vi "validate.vi"(8 "error in":errorcluster, 11 "Digitizer configuration":refnum<class "Digitizer configuration.lvclass">) -> (0 "error out":errorcluster, 3 "Digitizer configuration out":refnum<class "Digitizer configuration.lvclass">)   [LabVIEW 2025, in "Digitizer.lvlib" / "Digitizer configuration.lvclass"]
doc: "Provides an interface for performing validation on a given configuration. Any children should define the behavior of this function to ensure that the configuration in memory can be used by the runtime class.Copyright 2017 National Instruments Corporation\n\nLicensed under the Apache License, Version 2.0 (the \"License\"); you may not use this file except in compliance with the License. You may obtain a copy of the License at http://www.apache.org/licenses/LICENSE-2.0\nUnless required by applicable law or agreed to in writing, software distributed under the License is distributed on an \"AS IS\" BASIS, WITHOUT WARRANTIES OR CONDITIONS OF ANY KIND, either express or implied. See the License for the specific language governing permissions and limitations under the License."
uses:
  Digitizer configuration.lvclass
  Users/Public/Documents/Sandia National Labs/TSS Plugin/Abstract Engine.lvlibp/Plugin/Abstract/Instrument configuration/Read Instrument Setting.vi
  Digitizer configuration.lvclass/Digitizer configuration.ctl
  Users/Public/Documents/Sandia National Labs/TSS Plugin/CEF.lvlibp
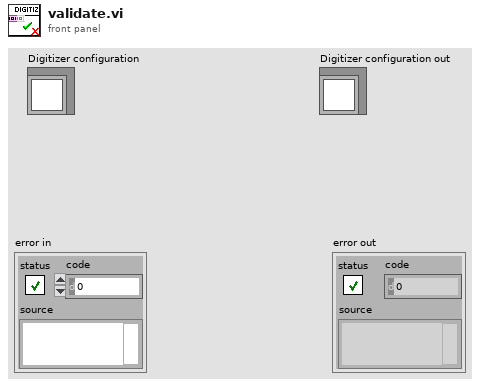
[diagram p1: front panel]
types:
  T1 = cluster{"Type":string, "Engine IP Address":string, "Engine Port":u32, "Address":string, "SW Alias":string, "Description":string, "Enabled":bool, "Model":string, "Serial Number":string, "Asset Number":string, "Calibration Date":string}
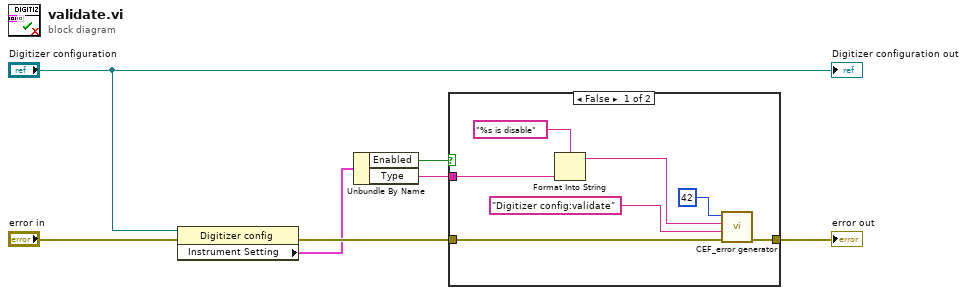
[diagram p0: block diagram]
diagram:
  n1 = property class="Digitizer config"(reference="Digitizer configuration", error in="error in") -> (error out=w3:errorcluster, "Instrument Setting"=w1:T1)  [unwired: 1 out]
  n2 = Unbundle By Name(w1) -> ("Enabled"=w5:bool, "Type"=w4:string)
  n3 = case shown="False" w5 {
    tunnel: w3 -> [w14 w15]
    tunnel: [w13 w15] -> w6
    tunnel: w4 -> [w10 _]
    frame False {
      n4 = Format Into String(format string="%s is disable" ("append error message"), w10) -> (resulting string=w9:string)  [unwired: 2 in, 1 out]
      n5 = call "CEF_error generator.vi"("error in"=w14, "source"="Digitizer config:validate", "append error message"=w9, "error code (0)"=42) -> ("error out"=w13:errorcluster)  [unwired: 5 in]
    }
    frame True {
    }
  }
  "error out" <- w6
  "Digitizer configuration out" <- "Digitizer configuration"
